vi "projekt 3.vi"() -> ()   [LabVIEW 2017]
panel:
  in  "F/C":bool
  in  "time":dbl
  in  "stop":bool
  out "C":dbl
  out "F":dbl
  out "temp C":dbl(slide) scale=0.0..100.0
  in  "temp F":dbl(slide) scale=0.0..200.0
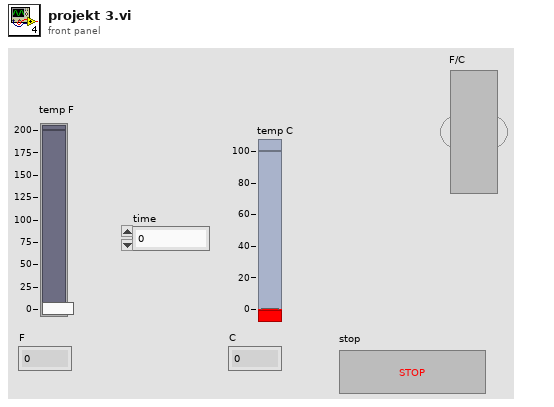
[diagram p1: front panel]
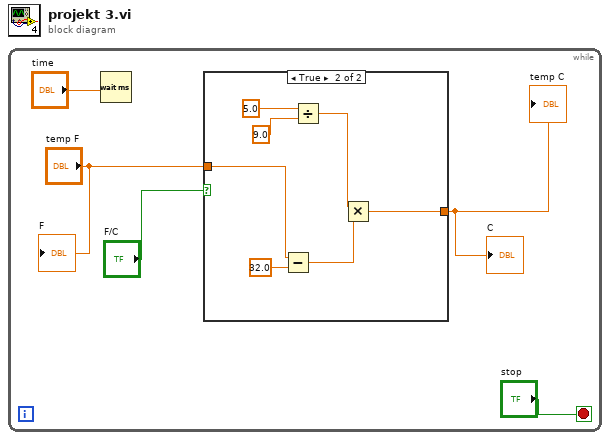
[diagram p0: block diagram]
diagram:
  n1 = while {
    stop <- "stop" stop-if-true
    n2 = Wait (ms)(milliseconds to wait="time") -> ()  [unwired: 1 out]
    n3 = case shown="True" "F/C" {
      tunnel: "temp F" -> [w6 w8]
      tunnel: [w6 w7] -> w1
      frame False {
      }
      frame True {
        n4 = Subtract(x=w8, y=32.0) -> (x-y=w12:dbl)
        n5 = Divide(x=5.0, y=9.0 ("x/y")) -> (x/y=w13:dbl)
        n6 = Multiply(x=w13, y=w12) -> (x*y=w7:dbl)
      }
    }
    "temp C" <- w1
    "C" <- w1
    "F" <- "temp F"
  }
